vi "Create All Real-Time Message Queues.vi"(8 "error in (no error)":errorcluster caption="错误输入（无错误）") -> (0 "error out":errorcluster caption="错误输出", 3 "Message Queues out":T1 caption="消息队列输出")   [LabVIEW 2013, in "Message Queue.lvlib"]
doc: "本VI用于创建应用程序所需的所有消息队列。如应用程序需要两个以上消息队列，可右键单击上面的“消息队列”常量并选择“打开自定义类型”，将新的消息队列添加至该自定义类型，然后通过本VI进行初始化。"
uses:
  Message Queue.lvlib
  All Real-Time Message Queues.ctl
  Message Cluster.ctl
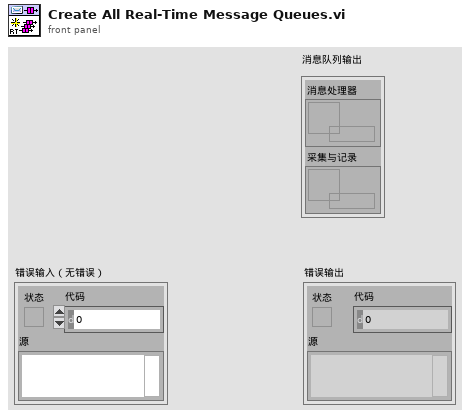
[diagram p1: front panel]
types:
  T1 = typedef "Message Queue.lvlib/All Real-Time Message Queues.ctl" = cluster{"Message Handler":refnum<queue>, "Acquisition and Logging":refnum<queue>}
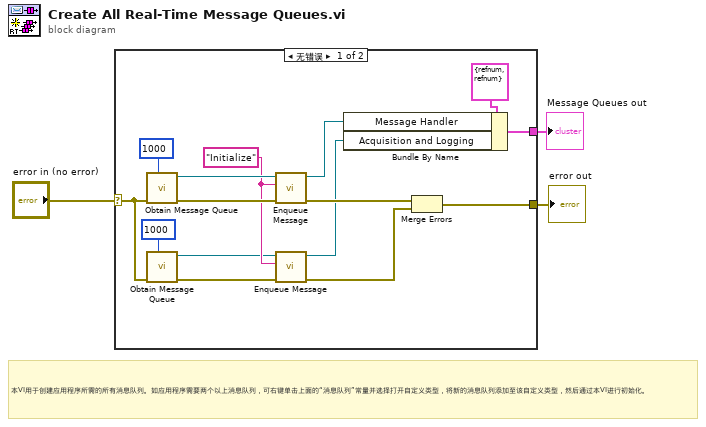
[diagram p0: block diagram]
diagram:
  # "本VI用于创建应用程序所需的所有消息队列。如应用程序需要两个以上消息队列，可右键单击上面的“消息队列”常量并选择打开自定义类型，将新的消息队列添加至该自定义类型，然后通过本VI进行初始化。"
  n1 = case shown="无错误" "error in (no error)" {
    selector: "error in (no error)" -> [w10 w19]
    tunnel: [w12 w19] -> w3
    tunnel: [w16 _] -> w2
    frame No Error {
      w8 = "Initialize" ("Message")
      n2 = call "Obtain Message Queue.vi"("max queue size (-1, unlimited)"=1000, "error in (no error)"=w10) -> ("error out"=w15:errorcluster, "Message Queue"=w14:refnum<queue>)  [unwired: 8 in]
      n3 = call "Obtain Message Queue.vi"("max queue size (-1, unlimited)"=1000, "error in (no error)"=w10) -> ("error out"=w11:errorcluster, "Message Queue"=w7:refnum<queue>)  [unwired: 8 in]
      n4 = call "Enqueue Message.vi"("error in (no error)"=w15, "Message"=w8, "Message Queue"=w14) -> ("error out"=w18:errorcluster, "dup Message Queue"=w13:refnum<queue>)  [unwired: 7 in]
      n5 = call "Enqueue Message.vi"("error in (no error)"=w11, "Message"=w8, "Message Queue"=w7) -> ("error out"=w9:errorcluster, "dup Message Queue"=w6:refnum<queue>)  [unwired: 7 in]
      n6 = Bundle By Name(cluster=T1 {"Message Handler"=refnum, "Acquisition and Logging"=refnum} ("Message Queues"), "Message Handler"=w13, "Acquisition and Logging"=w6) -> (w16:T1)
      n7 = Merge Errors(w18, w9) -> (w12:errorcluster)
    }
    frame Error {
    }
  }
  "Message Queues out" <- w2
  "error out" <- w3
